vi "Load Signal Bank (no wait).vi"(5 "Active AO Array":i32[](array[numeric]), 7 "Input array":dbl[][](array[numeric])=array10000x1[10000 elements] format="%.2f", 11 "error in (no error)":errorcluster) -> (15 "error out":errorcluster)   [LabVIEW 2015]
panel:
  out "Waveform Graph":dbl[][](graph)
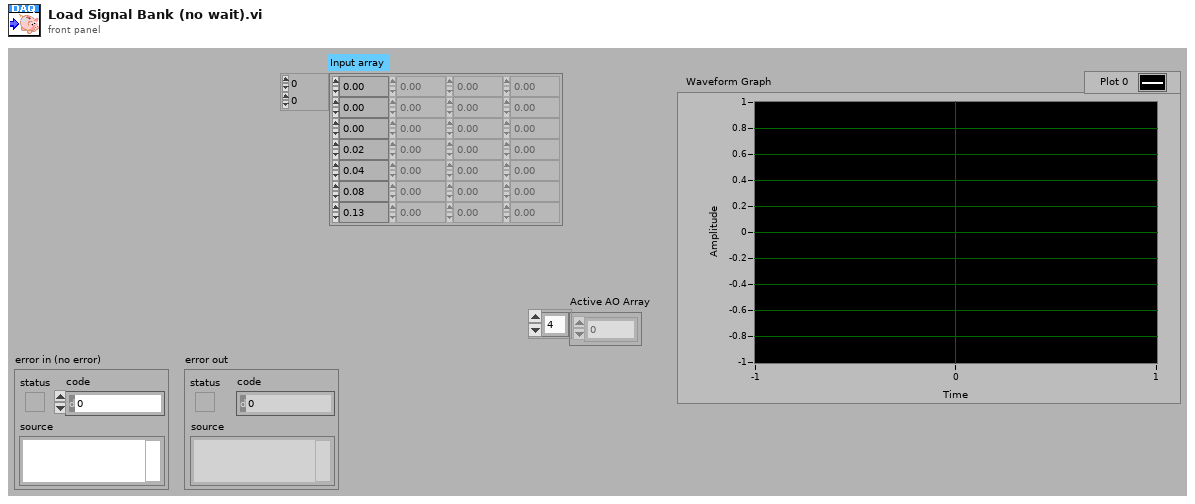
[diagram p1: front panel]
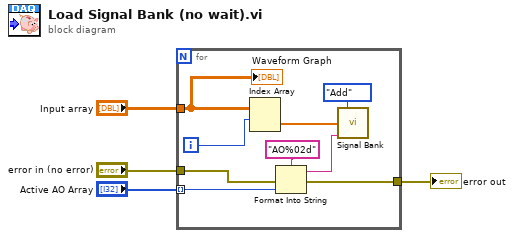
[diagram p0: block diagram]
diagram:
  n1 = for {
    tunnel: "Active AO Array" -> [w12] mode=indexing
    tunnel: "Input array" -> [w5]
    tunnel: "error in (no error)" -> [w7]
    tunnel: [w6] -> w1
    i -> [w10]
    n2 = Index Array(array=w5, index (row)=w10) -> (element=w9:dbl[])  [unwired: 1 in]
    n3 = Format Into String(format string="AO%02d", error in=w7, w12) -> (resulting string=w11:string, error out=w6:errorcluster)  [unwired: 1 in]
    n4 = call "Signal Bank.vi"("Action"=enum16{"Add", "Replace ID", "Read ID", "Clear"}."Add", "1D Data In"=w9, "ID"=w11) -> ()  [unwired: 11 in, 2 out]
    "Waveform Graph" <- w5
  }
  "error out" <- w1
